vi "GEN2_All_Error.vi"   [LabVIEW 2016, in "GEN_2.lvlib"]
uses:
  GEN_2.lvlib
  <vilib>/Utility/error.llb/Error Cluster From Error Code.vi
  <vilib>/ErrorRing/Error Ring.xnode
  <vilib>/Utility/error.llb/DialogType.ctl
types:
  T1 = typedef "DialogType.ctl" = u16
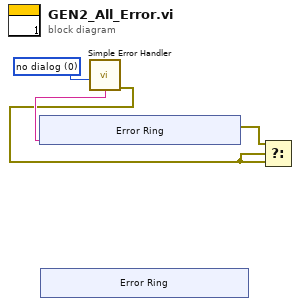
[diagram p0: block diagram]
diagram:
  w3 = T1 0 items=["no dialog", "OK message", "continue or stop message", "OK message + warnings", "continue/stop + warnings"] ("type of dialog (OK msg:1)")
  n1 = xnode "Error Ring"() -> ()  [unwired: 1 in, 1 out]
  n2 = call <vilib>:"Simple Error Handler.vi"("type of dialog (OK msg:1)"=w3) -> ("error out"=w1:errorcluster, "message"=w2:string)  [unwired: 4 in, 3 out]
  n3 = xnode "Error Ring"("parameter 0"=w2) -> ("error out"=w4:errorcluster)
  n4 = Select(t=w4, s=w1, f=w1) -> ()  [unwired: 1 out]
